vi "Initiate nodes.vi"(2 "Inputs":i8, 3 "X":i8) -> (0 "Y":i8[](array[numeric]), 1 "X":i8[](array[numeric]))   [LabVIEW 2010]
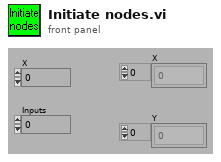
[diagram p1: front panel]
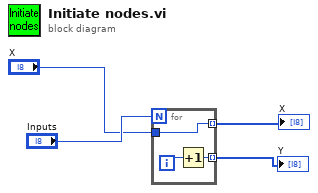
[diagram p0: block diagram]
diagram:
  n1 = for {
    N: "Inputs" -> [_]
    tunnel: [w6] -> w4 mode=indexing
    tunnel: [w5] -> w3 mode=indexing
    tunnel: "X" -> [w5]
    i -> [w7]
    n2 = Increment(x=w7) -> (x+1=w6:i32)
  }
  "Y" <- w4
  "X" <- w3
